vi "WPI_IMU_Loop.vi"(8 "error in":errorcluster, 11 "ADI IMU Interrupt DevRef":T1={"SimpleGyroDevRef"={"DevStatus"={"status"=FALSE, "code"=0, "source"=""}, "Handle"=0, "SPI Bus"=enum."SPI On-Board, CS0", "Device Found"=FALSE, "Sample Rate"=0.0, "Device Ready"=FALSE, "Yaw Axis"=enum."Z", "AHRS Algorithm"=enum."Complementary"}, "InterruptRef"={"DevStatus"={"status"=FALSE, "code"=0, "source"=""}, "InterruptIndex"=enum."0"}} {"SimpleGyroDevRef"."Sample Rate" min=0.25 max=100.0 step=0.25}) -> (0 "error out":errorcluster, 1 "Device Found":bool)   [LabVIEW 2015, in "FRC ADI MXP IMU.lvlib"]
doc: "Periodically reads the ADI MXP IMU valuse and makes data available for use elsewhere in your robot project. Place this block within PeriodicTasks.vi outside any loops."
uses:
  FRC ADI MXP IMU.lvlib
  WPI_AnalogDevicesIMUInterruptDevRef.ctl
  WPI_AnalogDevicesIMUDevRef.ctl
  <vilib>/Rock Robotics/SystemInterfaces/spilib/spi_bus.ctl
  <vilib>/Rock Robotics/WPI/Interrupt/WPI_InterruptRef.ctl
  <vilib>/Rock Robotics/SystemInterfaces/Interrupt/FPGA_InterruptIndex.ctl
  <vilib>/Rock Robotics/WPI/SPI/WPI_SPIDevRef.ctl
  <vilib>/Platform/TimedLoop/XDataNode/timing_clust.ctl
  <vilib>/Platform/TimedLoop/XDataNode/nitl_modes.ctl
  <vilib>/Platform/TimedLoop/XDataNode/wakeup.ctl
  <vilib>/Analysis/baseanly.llb/Mean (DBL).vi
  <vilib>/Rock Robotics/SystemInterfaces/Utilities/FPGA_UtilitiesRead LocalTime.vi
  <vilib>/Rock Robotics/SystemInterfaces/Interrupt/FPGA_WaitOnInterrupt.vi
  <vilib>/Rock Robotics/WPI/Utilities/WPI_UtilitiesTimebaseConstants.vi
  <vilib>/Rock Robotics/SystemInterfaces/Interrupt/FPGA_InterruptReadTimestamp.vi
  <vilib>/platform/TimedLoop/XDataNode/XDataNode.xnode
  <vilib>/Platform/TimedLoop/XDataNode/XDNodeRunTimeDep.lvlib
  <vilib>/Analysis/NI_AALBase.lvlib
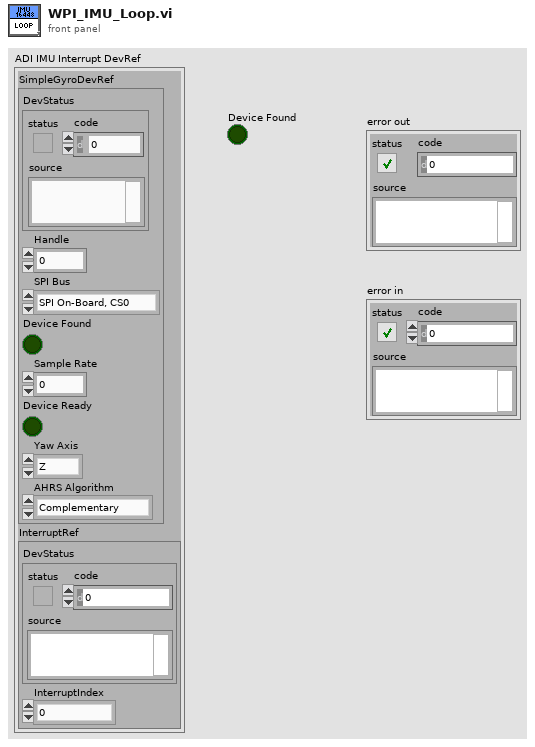
[diagram p1: front panel]
types:
  T1 = typedef "FRC ADI MXP IMU.lvlib/WPI_AnalogDevicesIMUInterruptDevRef.ctl" = cluster{"SimpleGyroDevRef":T2, "InterruptRef":T4}
  T2 = typedef "FRC ADI MXP IMU.lvlib/WPI_AnalogDevicesIMUDevRef.ctl" = cluster{"DevStatus":errorcluster, "Handle":i32, "SPI Bus":T3, "Device Found":bool, "Sample Rate":dbl, "Device Ready":bool, "Yaw Axis":enum16{"X", "Y", "Z"}, "AHRS Algorithm":enum16{"Complementary", "Madgwick"}}
  T3 = typedef "spi_bus.ctl" = enum16{"SPI On-Board, CS0", "SPI On-Board, CS1", "SPI On-Board, CS2", "SPI On-Board, CS3", "SPI MXP", "Invalid"}
  T4 = typedef "WPI_InterruptRef.ctl" = cluster{"DevStatus":errorcluster, "InterruptIndex":T5}
  T5 = typedef "FPGA_InterruptIndex.ctl" = enum8{"0", "1", "2", "3", "4", "5", "6", "7", "Invalid"}
  T6 = typedef "WPI_SPIDevRef.ctl" = cluster{"DevStatus":errorcluster, "Handle":i32, "SPI Bus":T3}
  T7 = cluster{"X Angle":dbl, "Y Angle":dbl, "Z Angle":dbl}
  T8 = typedef "XDNodeRunTimeDep.lvlib/timing_clust.ctl" = cluster{"Expected End [f-1]":u64, "Actual End [f-1]":u64, "Finished Late? [f-1]":bool, "Expected End [i-1]":u64, "Actual End [i-1]":u64, "Finished Late? [i-1]":bool, "Expected Start [i]":u64, "Actual Start [i]":u64, "Expected Start [f]":u64, "Actual Start [f]":u64, "Source Name":string, "Structure Name":string, "Period":i64, "Deadline":i64, "Offset":i64, "Start":i64, "Priority":i32, "Timeout":i32, "Mode":T9, "Wakeup Reason":T10, "Error":errorcluster, "Source Type":string, "Secondary Source Type":string, "Global End Time":u64, "Global Start Time":u64, "Frame Duration":u64, "Iteration Duration":u64, "Assigned CPU":i32, "I/O Scan Engine Mode":u32}
  T9 = typedef "XDNodeRunTimeDep.lvlib/nitl_modes.ctl" = enum32{"No Change", "Process missed periods, maintain original phase", "Discard missed periods, maintain original phase", "Process missed periods, ignore original phase", "Discard missed periods, ignore original phase"}
  T10 = typedef "XDNodeRunTimeDep.lvlib/wakeup.ctl" = enum32{"Normal", "Aborted", "Asynchronous wakeup", "Timing source error", "Timed loop error", "Timeout"}
  T11 = cluster{"Output[0]":dbl, "Output[1]":dbl, "Output[2]":dbl}
  T12 = cluster{"Data Array[0]":dbl, "Data Array[1]":dbl, "Data Array[2]":dbl, "Data Array[3]":dbl, "Data Array[4]":dbl, "Data Array[5]":dbl, "Data Array[6]":dbl, "Data Array[7]":dbl, "Data Array[8]":dbl, "Data Array[9]":dbl, "Data Array[10]":dbl}
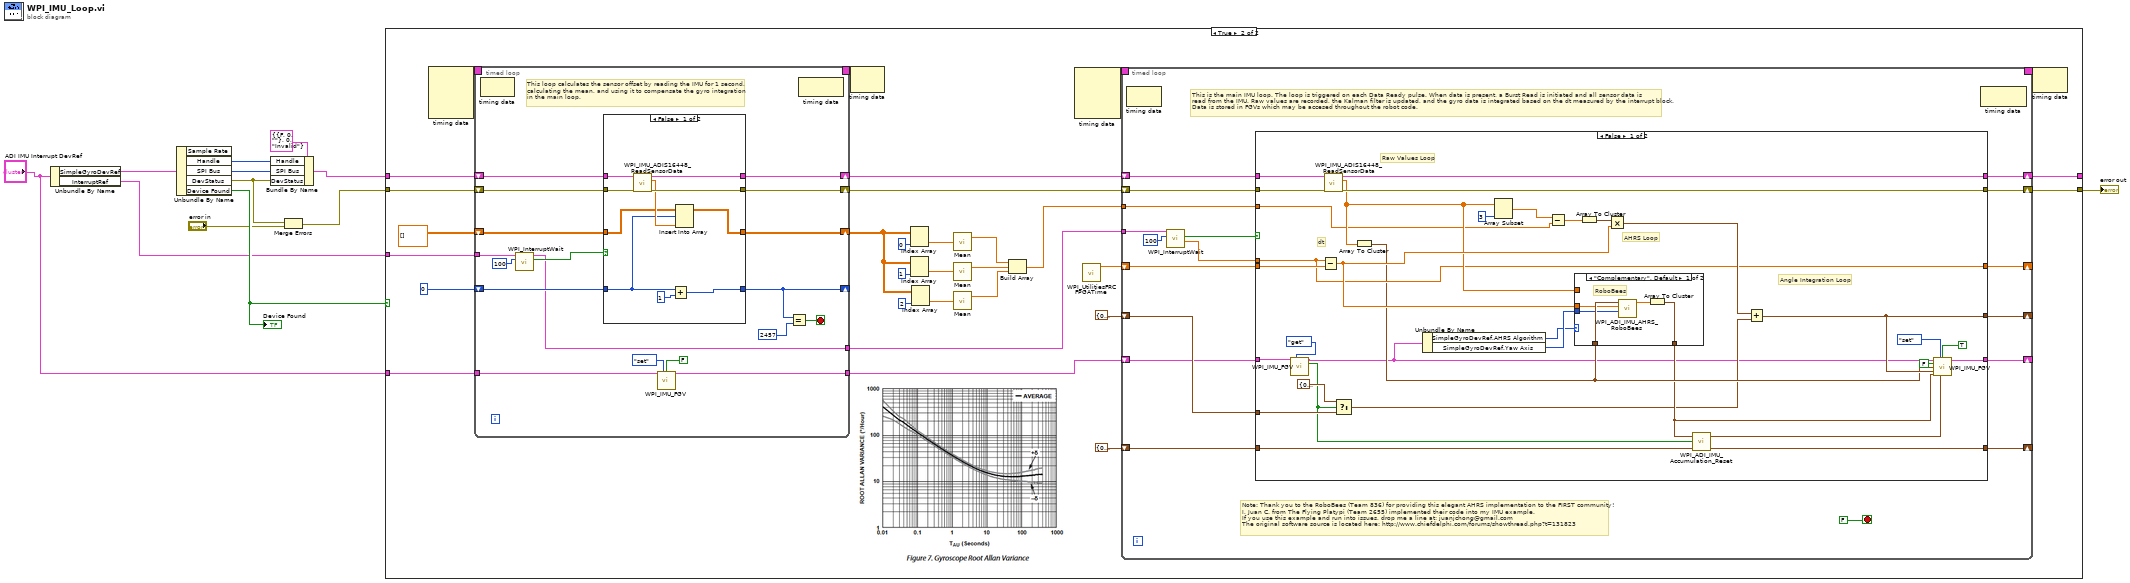
[diagram p0: block diagram]
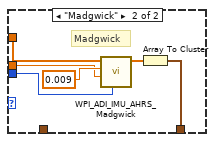
[diagram p4: hidden frame]
diagram:
  n1 = Unbundle By Name("ADI IMU Interrupt DevRef") -> ("SimpleGyroDevRef"=w6:T2, "InterruptRef"=w5:T4)
  n2 = Unbundle By Name(w6) -> ("Handle"=w11:i32, "SPI Bus"=w10:T3, "DevStatus"=w3:errorcluster, "Device Found"=w9:bool)  [unwired: 1 out]
  "Device Found" <- w9
  n3 = Bundle By Name(cluster=T6 {"DevStatus"={"status"=FALSE, "code"=0, "source"=""}, "Handle"=0, "SPI Bus"=enum."Invalid"} ("SPIDevRef out"), "Handle"=w11, "SPI Bus"=w10, "DevStatus"=w3) -> (w8:T6)
  n4 = Merge Errors(w3, "error in") -> (w1:errorcluster)
  n5 = case shown="True" w9 {
    tunnel: w8 -> [w14 w34]
    tunnel: w1 -> [w13 w33]
    tunnel: [w13 w44] -> w7
    tunnel: [w14 w43] -> _
    tunnel: "ADI IMU Interrupt DevRef" -> [_ w31]
    tunnel: w5 -> [_ w32]
    frame False {
    }
    frame True {
      n6 = node-c288() -> (w38:T8)  [unwired: 4 in]
      n7 = timed-loop {
        shift-right: [w61] -> w36
        shift-left: w34 -> [w55]
        shift-right: [w62] -> w35
        shift-left: w33 -> [w54]
        shift-right: [w46] -> _
        shift-left: 0 -> [w59]
        tunnel: w32 -> [w58]
        tunnel: [w53] -> w29
        timing: w38 -> [_]
        timing-out: [_] -> w37
        tunnel: w31 -> [w51]
        tunnel: [w52] -> w30
        shift-right: [w60] -> w23
        shift-left: dbl[][] [] -> [w48]
        stop <- w45 stop-if-true
        # "This loop calculates the sensor offset by reading the IMU for 1 second, \ncalculating the mean, and using it to compensate the gyro integration\nin the main loop."
        n8 = node-c288() -> ()  [unwired: 1 in, 1 out]
        n9 = call <vilib>:"WPI_InterruptWait.vi"("Timeout (ms)"=100, "InterruptRef"=w58) -> ("Timed Out"=w56:bool, "InterruptRef"=w53:T4)  [unwired: 5 in, 3 out]
        n10 = case shown="False" w56 {
          tunnel: [w74 w76] -> w62
          tunnel: [w73 w77] -> w61
          tunnel: [w65 w75] -> w60
          tunnel: w54 -> [w72 w76]
          tunnel: w55 -> [w71 w77]
          tunnel: w59 -> [w66 w78]
          tunnel: [w70 w78] -> w46
          tunnel: w48 -> [w67 w75]
          frame False {
            n11 = call "WPI_IMU_ADIS16448_ReadSensorData.vi"("error in (no error)"=w72, "SPIDevRef in"=w71) -> ("error out"=w74:errorcluster, "Data Array"=w68:dbl[], "SPIDevRef out"=w73:T6)  [unwired: 7 in]
            n12 = Add(x=w66, y=1) -> (x+y=w70:i32)
            n13 = Insert Into Array(array=w67, index (row)=w66, new element=w68) -> (w65:dbl[][])  [unwired: 1 in]
          }
          frame True {
          }
        }
        n14 = call "WPI_IMU_FGV.vi"("ADI IMU Interrupt DevRef"=w51, "Operation"=enum16{"set", "get"}."set", "Sensor Ready?"=FALSE) -> ("ADI IMU Interrupt DevRef Out"=w52:T1)  [unwired: 6 in, 6 out]
        n15 = Equal?(x=w46, y=2457) -> (x = y?=w45:bool)
        n16 = node-c288() -> ()  [unwired: 1 in, 1 out]
      }
      n17 = node-c288(w37) -> ()  [unwired: 1 out]
      n18 = Index Array(array=w23, index (col)=0 ("disabled index (col)")) -> (element=w22:dbl[])  [unwired: 1 in]
      n19 = Index Array(array=w23, index (col)=1 ("disabled index (col)")) -> (element=w21:dbl[])  [unwired: 1 in]
      n20 = Index Array(array=w23, index (col)=2 ("disabled index (col)")) -> (element=w20:dbl[])  [unwired: 1 in]
      n21 = call-poly <vilib>:"Mean.vi"("X"=w22) -> ("mean"=w19:dbl)  [unwired: 1 out]
      n22 = call-poly <vilib>:"Mean.vi"("X"=w21) -> ("mean"=w18:dbl)  [unwired: 1 out]
      n23 = call-poly <vilib>:"Mean.vi"("X"=w20) -> ("mean"=w17:dbl)  [unwired: 1 out]
      n24 = Build Array(w19, w18, w17) -> (w16:dbl[])
      n25 = node-c288() -> (w41:T8)  [unwired: 4 in]
      n26 = call <vilib>:"WPI_UtilitiesFRC FPGATime.vi"() -> ("FPGA Time"=w15:dbl)  [unwired: 10 in, 1 out]
      n27 = timed-loop {
        shift-right: [w98] -> w43
        shift-left: w36 -> [w94]
        shift-right: [w97] -> w44
        shift-left: w35 -> [w93]
        shift-right: [w95] -> _
        shift-left: cluster{dbl, dbl, dbl} {0.0, 0.0, 0.0} -> [w82]
        tunnel: w29 -> [w91]
        shift-right: [w87] -> _
        shift-left: w15 -> [w89]
        timing: w41 -> [_]
        timing-out: [_] -> w40
        shift-right: [w85] -> _
        shift-left: T7 {"X Angle"=0.0, "Y Angle"=0.0, "Z Angle"=0.0} ("input cluster") -> [w86]
        tunnel: w16 -> [w84]
        shift-right: [w83] -> _
        shift-left: w30 -> [w81]
        stop <- FALSE stop-if-true
        # "Note: Thank you to the RoboBees (Team 836) for providing this elegant AHRS implementation to the FIRST community!\nI, Juan C. from The Flying Platypi (Team 2655) implemented their code into my IMU example.\nIf you use this example and run into issues, drop me a line at: juanjchong@gmail.com\nThe original software source is located here: http://www.chiefdelphi.com/forums/showthread.php?t=131823"
        # "This is the main IMU loop. The loop is triggered on each Data Ready pulse. When data is present, a Burst Read is initiated and all sensor data is \nread from the IMU. Raw values are recorded, the Kalman filter is updated, and the gyro data is integrated based on the dt measured by the interrupt block.\nData is stored in FGVs which may be accesed throughout the robot code."
        n28 = node-c288() -> ()  [unwired: 1 in, 1 out]
        n29 = call <vilib>:"WPI_InterruptWait.vi"("Timeout (ms)"=100, "InterruptRef"=w91) -> ("TimeStamp"=w90:dbl, "Timed Out"=w88:bool)  [unwired: 5 in, 3 out]
        n30 = case shown="False" w88 {
          tunnel: w94 -> [w133 w150]
          tunnel: w93 -> [w132 w149]
          tunnel: [w131 w150] -> w98
          tunnel: [w130 w149] -> w97
          tunnel: [w118 w145] -> w95
          tunnel: w90 -> [w119 _]
          tunnel: w89 -> [w125 w148]
          tunnel: [w119 w148] -> w87
          tunnel: w86 -> [w113 w147]
          tunnel: [w114 w147] -> w85
          tunnel: w84 -> [w110 _]
          tunnel: w81 -> [w104 w146]
          tunnel: [w109 w146] -> w83
          tunnel: w82 -> [w105 w145]
          frame False {
            # "dt"
            # "Angle Integration Loop"
            # "AHRS Loop"
            # "Raw Values Loop"
            n31 = call "WPI_IMU_FGV.vi"("ADI IMU Interrupt DevRef"=w104, "Operation"=enum16{"set", "get"}."get") -> ("ADI IMU Interrupt DevRef Out"=w103:T1, "Reset Out"=w101:bool)  [unwired: 7 in, 5 out]
            n32 = Subtract(x=w119, y=w125) -> (x-y=w123:dbl)
            n33 = call "WPI_IMU_ADIS16448_ReadSensorData.vi"("error in (no error)"=w132, "SPIDevRef in"=w133) -> ("error out"=w130:errorcluster, "Data Array"=w121:dbl[], "SPIDevRef out"=w131:T6)  [unwired: 7 in]
            n34 = Select(t=T11 {"Output[0]"=0.0, "Output[1]"=0.0, "Output[2]"=0.0} ("cluster"), s=w101, f=w105) -> (s? t:f=w106:T11)
            n35 = Array To Cluster(array=w121) -> (cluster=w117:T12)
            n36 = Unbundle By Name(w103) -> ("SimpleGyroDevRef.AHRS Algorithm"=w120:enum16{"Complementary", "Madgwick"}, "SimpleGyroDevRef.Yaw Axis"=w122:enum16{"X", "Y", "Z"})
            n37 = Array Subset(array=w121, length=3) -> (w112:dbl[])  [unwired: 1 in]
            n38 = Subtract(x=w112, y=w110) -> (x-y=w111:dbl[])
            n39 = case shown="\"Complementary\", Default" w120 {
              tunnel: [w137 w142] -> w116
              tunnel: w117 -> [w136 _]
              tunnel: w123 -> [w135 w141]
              tunnel: w122 -> [w134 w139]
              tunnel: w121 -> [_ w140]
              frame "Complementary", Default {
                # "RoboBees"
                n40 = call "WPI_ADI_IMU_AHRS_RoboBees.vi"("Yaw Axis"=w134, "dt (s)"=w135, "IMU Rates"=w136) -> ("Output"=w138:dbl[])  [unwired: 4 in, 3 out]
                n41 = Array To Cluster(array=w138) -> (cluster=w137:T11)
              }
              frame "Madgwick" {
                # "Madgwick"
                n42 = call "WPI_ADI_IMU_AHRS_Madgwick.vi"("Yaw Axis"=w139, "dt (s)"=w141, "Beta"=0.009, "Data"=w140) -> ("Output"=w143:dbl[])  [unwired: 7 in]
                n43 = Array To Cluster(array=w143) -> (cluster=w142:T11)
              }
            }
            n44 = Array To Cluster(array=w111) -> (cluster=w127:cluster{"[0]":dbl, "[1]":dbl, "[2]":dbl})
            n45 = Multiply(x=w127, y=w123) -> (x*y=w126:cluster{"[0]":dbl, "[1]":dbl, "[2]":dbl})
            n46 = call "WPI_ADI_IMU_Accumulation_Reset.vi"("AHRS Reset In"=w113, "Reset?"=w101, "Absolute Angle In"=w116) -> ("AHRS Reset Out"=w114:T7, "Converted Output"=w115:T11)  [unwired: 1 in]
            n47 = Add(x=w126, y=w106) -> (x+y=w118:cluster{dbl, dbl, dbl})
            n48 = call "WPI_IMU_FGV.vi"("ADI IMU Interrupt DevRef"=w103, "Operation"=enum16{"set", "get"}."set", "Sensor Ready?"=TRUE, "Reset"=FALSE, "IMU Data"=w117, "IMU Angles"=w118, "IMU AHRS"=w116, "IMU AHRS DELTA"=w115) -> ("ADI IMU Interrupt DevRef Out"=w109:T1)  [unwired: 1 in, 6 out]
          }
          frame True {
            # "Waiting for an interrupt..."
          }
        }
        n49 = node-c288() -> ()  [unwired: 1 in, 1 out]
      }
      n50 = node-c288(w40) -> ()  [unwired: 1 out]
    }
  }
  "error out" <- w7
